vi "USB Relay Control.vi"   [LabVIEW 2019]
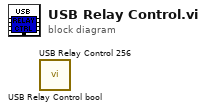
[diagram p0: block diagram]
diagram:
  n1 = call "USB Relay Control bool.vi"() -> ()  [unwired: 11 in, 1 out]
  n2 = call "USB Relay Control 256.vi"() -> ()  [unwired: 11 in, 1 out]
